vi "Cannon Problem Fix.vi"(1 "Cannon Global Data Modified":T2, 2 "Cannon Global Data Original":T2) -> (0 "Cannon Global Data New":T2)   [LabVIEW 2013]
uses:
  <vilib>/Rock Robotics/WPI/Solenoid/WPI_SolenoidValue.ctl
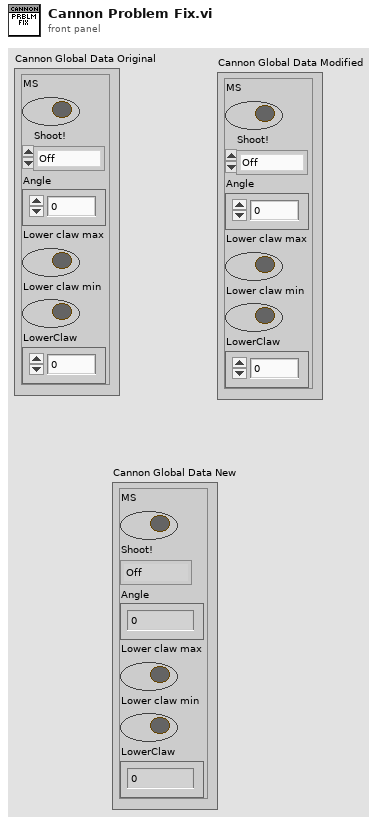
[diagram p1: front panel]
types:
  T1 = typedef "WPI_SolenoidValue.ctl" = enum16{"Off", "On", "Forward", "Reverse"}
  T2 = cluster{"MS":bool, "Shoot!":T1, "Angle":dbl, "Lower claw max":bool, "Lower claw min":bool, "LowerClaw":dbl}
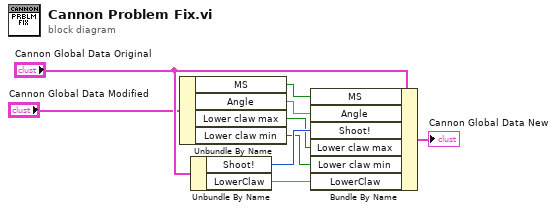
[diagram p0: block diagram]
diagram:
  n1 = Unbundle By Name("Cannon Global Data Modified") -> ("MS"=w6:bool, "Angle"=w5:dbl, "Lower claw max"=w3:bool, "Lower claw min"=w2:bool)
  n2 = Unbundle By Name("Cannon Global Data Original") -> ("Shoot!"=w4:T1, "LowerClaw"=w1:dbl)
  n3 = Bundle By Name(cluster="Cannon Global Data Original", "MS"=w6, "Angle"=w5, "Shoot!"=w4, "Lower claw max"=w3, "Lower claw min"=w2, "LowerClaw"=w1) -> (→"Cannon Global Data New":T2)
